vi "testAllWithXmlReport.vi"(8 "error in (no error)":errorcluster) -> (0 "error out":errorcluster)   [LabVIEW 2018]
doc: "Do all unit test and generate xml report."
uses:
  <vilib>/addons/_JKI Toolkits/Caraya/classes/Test Suite/Define Test Suite (JUnit Report).vi
  <vilib>/addons/_JKI Toolkits/Caraya/classes/Test Suite/Test Suite.lvclass
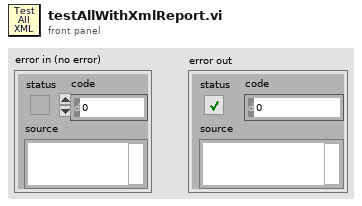
[diagram p1: front panel]
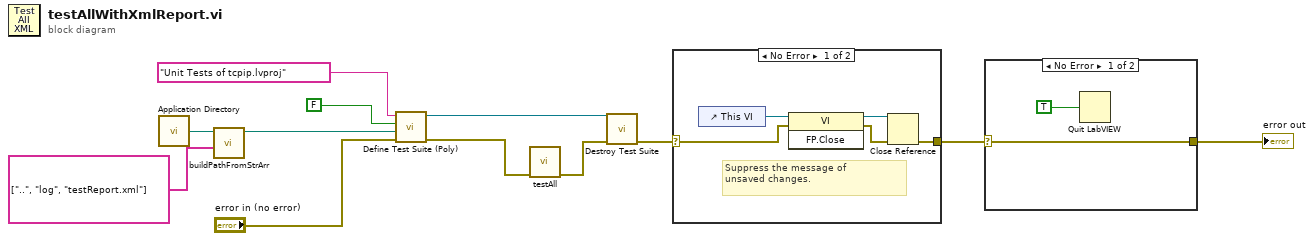
[diagram p0: block diagram]
diagram:
  n1 = call <vilib>:"Application Directory.vi"() -> ("Application Directory"=w2:path)
  n2 = call "buildPathFromStrArr.vi"("String Array"=string[] ["..", "log", "testReport.xml"], "Root Path"=w2) -> ("Absolute Path"=w1:path)  [unwired: 9 in]
  n3 = call-poly <vilib>:"Define Test Suite (Poly).vi"("error in (no error)"="error in (no error)", "Report Path"=w1, "Interactive"=FALSE, "Label (VI Title)"="Unit Tests of tcpip.lvproj") -> ("error out"=w7:errorcluster, "Test Suite"=w12:refnum<class "Test Suite.lvclass">)  [unwired: 6 in]
  n4 = call "testAll.vi"("error in (no error)"=w7) -> ("error out"=w6:errorcluster)  [unwired: 10 in]
  n5 = call-dynamic "Destroy Test Suite.vi"("error in (no error)"=w6, "Test Suite in"=w12) -> ("error out"=w9:errorcluster)  [unwired: 9 in]
  n6 = case shown="No Error" w9 {
    selector: w9 -> [w16 w18]
    tunnel: [w13 w18] -> w8
    frame No Error {
      # "Suppress the message of\nunsaved changes."
      n7 = control-ref of="This VI"() -> (w17:refnum<vi>)
      n8 = invoke class="VI" method="FP.Close"(reference=w17, error in=w16) -> (reference out=w15:refnum<vi>, error out=w14:errorcluster)  [unwired: 1 in, 1 out]
      n9 = Close Reference(reference=w15, error in (no error)=w14) -> (error out=w13:errorcluster)
    }
    frame Error {
    }
  }
  n10 = case shown="No Error" w8 {
    selector: w8 -> [w19 w21]
    tunnel: [w19 w21] -> w5
    frame No Error {
      n11 = Quit LabVIEW(quit? (T)=TRUE) -> ()
    }
    frame Error {
    }
  }
  "error out" <- w5
